vi "Run Vi.vi"(0 "Bring To Front (T)":bool=TRUE, 2 "VI Path":path, 3 "error in (no error)":errorcluster, 4 "Start Hidden? (F)":bool) -> (7 "Window State":T1(ring), 9 "error out":errorcluster)   [LabVIEW 2019]
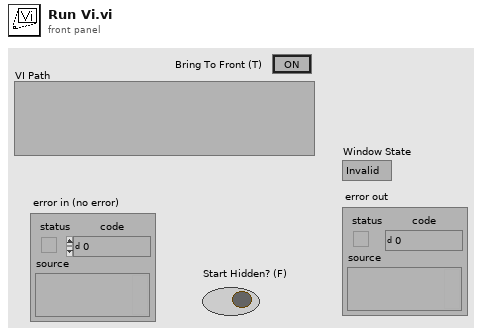
[diagram p1: front panel]
types:
  T1 = enum32{"Invalid", "Standard", "Closed", "Hidden", "Minimized", "Maximized"}
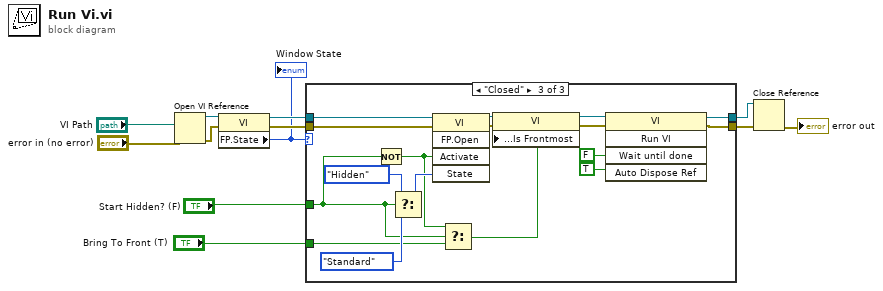
[diagram p0: block diagram]
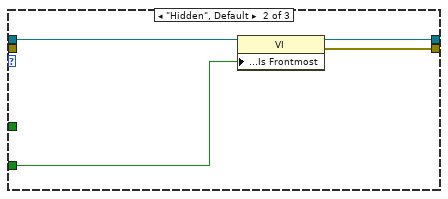
[diagram p3: hidden frame]
diagram:
  n1 = Open VI Reference(vi path="VI Path", error in (no error)="error in (no error)") -> (vi reference=w12:refnum<vi>, error out=w11:errorcluster)  [unwired: 4 in]
  n2 = property class="VI"(reference=w12, error in=w11) -> (reference out=w10:refnum<vi>, error out=w9:errorcluster, "FP.State"=w5:T1)
  "Window State" <- w5
  n3 = case shown="\"Closed\"" w5 {
    tunnel: w10 -> [w13 w18 w35]
    tunnel: w9 -> [w14 _ w27]
    tunnel: [w14 w17 w31] -> w3
    tunnel: "Bring To Front (T)" -> [_ w16 w22]
    tunnel: "Start Hidden? (F)" -> [_ _ w23]
    tunnel: [w13 w15 w19] -> w1
    frame "Invalid" {
    }
    frame "Hidden", Default {
      n4 = property class="VI"(reference=w18, "Front Panel Window:Is Frontmost"=w16) -> (reference out=w15:refnum<vi>, error out=w17:errorcluster)  [unwired: 1 in]
    }
    frame "Closed" {
      n5 = Not(x=w23) -> (.not. x?=w21:bool)
      n6 = Select(t=T1."Hidden" ("State"), s=w23, f=T1."Standard" ("State")) -> (s? t:f=w24:T1)
      n7 = invoke class="VI" method="FP.Open"(reference=w35, error in=w27, "Activate"=w21, "State"=w24) -> (reference out=w29:refnum<vi>, error out=w28:errorcluster)  [unwired: 1 in, 3 out]
      n8 = Select(t=w21, s=w23, f=w22) -> (s? t:f=w20:bool)
      n9 = property class="VI"(reference=w29, error in=w28, "Front Panel Window:Is Frontmost"=w20) -> (reference out=w34:refnum<vi>, error out=w33:errorcluster)
      n10 = invoke class="VI" method="Run VI"(reference=w34, error in=w33, "Wait until done"=FALSE, "Auto Dispose Ref"=TRUE) -> (reference out=w19:refnum<vi>, error out=w31:errorcluster)  [unwired: 1 in, 3 out]
    }
  }
  n11 = Close Reference(reference=w1, error in (no error)=w3) -> (error out=→"error out":errorcluster)
